vi "Main.vi"() -> ()   [LabVIEW 2015]
uses:
  <vilib>/NI/PowerElectronicsControl/BufferLogging/BufferConfig.ctl
  <vilib>/NI/PowerElectronicsControl/ScaleAndLimit/Interface/Configuration.ctl
  <vilib>/FPGAPlugInAG/sbRIO-9607/niLvFpga_Open_sbRIO-9607.vi
  <vilib>/rvi/interface/common/dynamic/niFpgaDynamicAddResources.vi
  <vilib>/FPGAPlugInAG/Dynamic/niLvFpga_Reset_Dynamic.vi
  <vilib>/FPGAPlugInAG/Dynamic/niLvFpga_Run_Dynamic.vi
  <vilib>/Utility/error.llb/Error Cluster From Error Code.vi
  <vilib>/rvi/errors/niLvFpgaAdjustHostInterfaceError.vi
  <vilib>/rvi/interface/nirviOpenFPGA/nirviOpenFPGA.xnode
  FPGA Bitfiles/BaseApplication_FPGATarget_Firmware_DvSj-lU7Yzc.lvbitx
  FPGA/Firmware.vi
  <vilib>/rvi/interface/nirviMethod/nirviMethod.xnode
  <vilib>/rvi/interface/nirviReadWriteControl/nirviReadWriteControl.xnode
  <instrlib>/_niInstr/FIFO Register Bus/v1/Host/niInstr FIFO Register Bus v1 Host.lvclass
  <vilib>/NI/PowerElectronicsControl/BufferLogging/BufferLogging.lvlib
  <instrlib>/_niInstr/Instruction Framework/v1/Host/Subsystem Map/niInstr Subsystem Map v1 Host.lvclass
  <vilib>/NI/PowerElectronicsControl/ScaleAndLimit/Interface/ScaleAndLimitInterface.lvlib
  <vilib>/NI/PowerElectronicsControl/WaveformAcq/IFw_Addon/RT/WaveformTask.lvclass
  NiFpgaLv.dll
  <vilib>/rvi/interface/Simulation/niFpgaSimulationCallBeginRW.vi
panel:
  out "AI Limits":string
  in  "UI Update Rate(s)":dbl=5.0 format="%#_13g"
  in  "TriggerLog":bool
  out "Waveforms":sgl[][](graph)
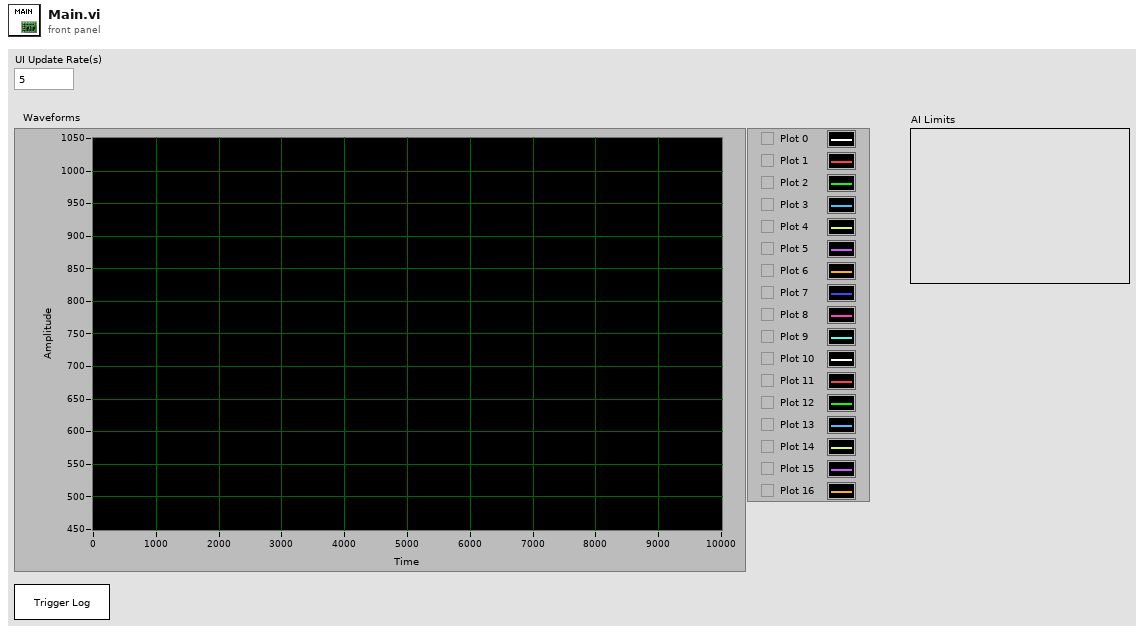
[diagram p1: front panel]
types:
  T1 = cluster{"Channel Name":string, "Sensitivity mV_EU":dbl, "EU":string, "dB Ref EU":dbl}
  T2 = typedef "BufferLogging.lvlib/BufferConfig.ctl" = cluster{"Channels":string[], "pretriggerTime_sec":dbl, "posttriggerTime_sec":dbl, "BlockSizePerChannel":i32, "SampleRate_Hz":dbl, "decimation factor":i32, "logDirectory":path, "logPrefix":string, "max files":i32}
  T3 = typedef "ScaleAndLimitInterface.lvlib/Configuration.ctl" = cluster{"Name":string, "M":dbl, "B":i16, "HighLimit":dbl, "LowLimit":dbl, "LimitsEnabled":bool}
  T4 = cluster{"Channel Name":string, "Sensitivity mV_EU":dbl, "EU":string, "dB Ref EU":dbl}[]
  T5 = typedef "BufferLogging.lvlib/Buffers.ctl" = cluster{"Channels":string[], "PosttriggerBuffer":refnum<queue>, "PretriggerBuffer":refnum<queue>, "BlockSizePerChannel":i32, " logging semaphore":T6, "Log refnum":refnum<k34>, "snapshotBuffer":refnum<data-value>, "logDirectory":path, "logPrefix":string, "decimation factor":i32, "max files":i32, "SampleRate":dbl}
  T6 = typedef "Semaphore RefNum" = refnum<k1>
  T7 = typedef "ScaleAndLimitInterface.lvlib/Interface.ctl" = cluster{"instruction target":refnum<class "niInstr Instruction Target v1 Host.lvclass">, "ScalingAndLimitsContext":refnum<class "niInstr Instruction Framework Context v1 Host.lvclass">, "Configuration":T3[]}
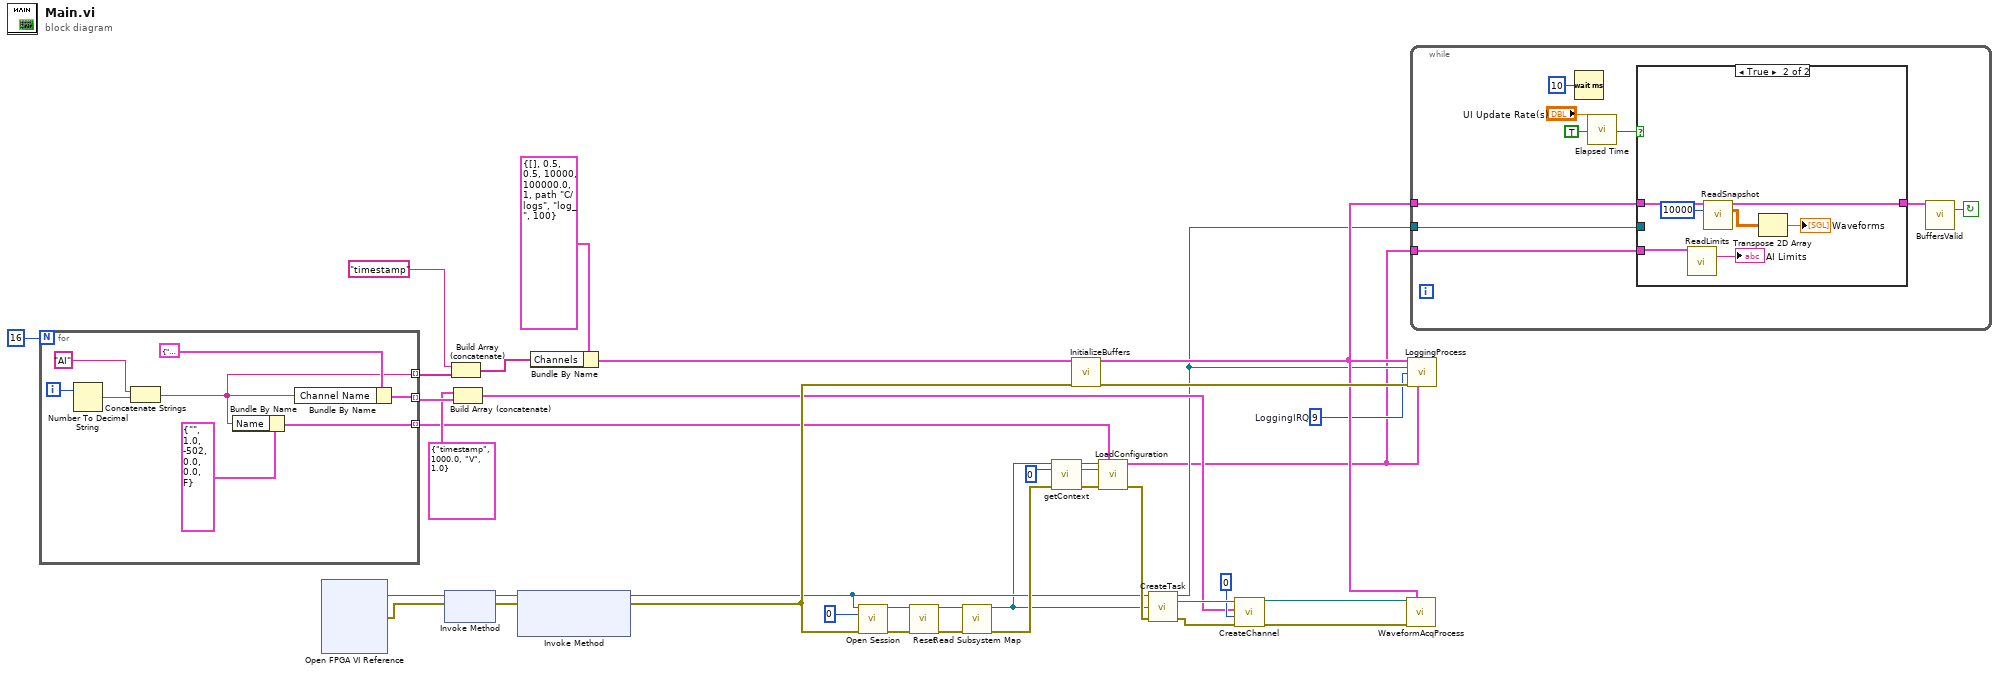
[diagram p0: block diagram]
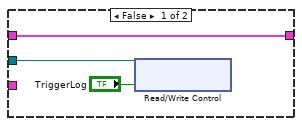
[diagram p2: hidden frame]
diagram:
  w2 = 9  # LoggingIRQ
  n1 = for {
    N: 16 -> [_]
    tunnel: [w40] -> w30 mode=indexing
    tunnel: [w42] -> w32 mode=indexing
    tunnel: [w39] -> w9 mode=indexing
    i -> [w46]
    n2 = Number To Decimal String(number=w46) -> (decimal integer string=w45:string)  [unwired: 1 in]
    n3 = Concatenate Strings("AI", w45) -> (w40:string)
    n4 = Bundle By Name(cluster=T3 {"Name"="", "M"=1.0, "B"=-502, "HighLimit"=0.0, "LowLimit"=0.0, "LimitsEnabled"=FALSE} ("Configuration"), "Name"=w40) -> (w39:T3)
    n5 = Bundle By Name(cluster=T1 {"Channel Name"="Untitled", "Sensitivity mV_EU"=1000.0, "EU"="V", "dB Ref EU"=1.0} ("Channel Info 2"), "Channel Name"=w40) -> (w42:T1)
  }
  n6 = xnode "Open FPGA VI Reference"() -> ("FPGA VI Reference Out"=w37:refnum<k20>, "error out"=w36:errorcluster)  [unwired: 2 in]
  n7 = xnode "Invoke Method"("FPGA VI Reference In"=w37, "error in"=w36) -> ("FPGA VI Reference Out"=w38:refnum<k20>, "error out"=w21:errorcluster)
  n8 = Build Array (concatenate)("timestamp", w30) -> (w28:string[])
  n9 = Build Array (concatenate)(T1 {"Channel Name"="timestamp", "Sensitivity mV_EU"=1000.0, "EU"="V", "dB Ref EU"=1.0} ("Channel Info 2"), w32) -> (w10:T4)
  n10 = xnode "Invoke Method"("FPGA VI Reference In"=w38, "error in"=w21) -> ("FPGA VI Reference Out"=w5:refnum<k20>, "error out"=w11:errorcluster)  [unwired: 1 in]
  n11 = Bundle By Name(cluster=T2 {"Channels"=[], "pretriggerTime_sec"=0.5, "posttriggerTime_sec"=0.5, "BlockSizePerChannel"=10000, "SampleRate_Hz"=100000.0, "decimation factor"=1, "logDirectory"=path "C:/logs", "logPrefix"="log_", "max files"=100} ("BufferConfig"), "Channels"=w28) -> (w34:T2)
  n12 = call <instrlib>:"Open Session.vi"("fpga ref"=w5, "bus instance"=u32 0, "error in"=w11) -> ("session out"=w24:refnum<class "niInstr FIFO Register Bus v1 Host.lvclass">, "error out"=w26:errorcluster)  [unwired: 11 in]
  n13 = call-dynamic "Reset.vi"("session in"=w24, "error in"=w26) -> ("session out"=w23:refnum<class "niInstr FIFO Register Bus v1 Host.lvclass">, "error out"=w22:errorcluster)  [unwired: 12 in]
  n14 = call <instrlib>:"Read Subsystem Map.vi"("instruction target in"=w23, "error in"=w22) -> ("instruction target out"=w4:refnum<class "niInstr FIFO Register Bus v1 Host.lvclass">, "error out"=w12:errorcluster)  [unwired: 11 in, 1 out]
  n15 = call <vilib>:"getContext.vi"("session in"=w4, "instance"=u8 0, "error in"=w12) -> ("session out"=w18:refnum<class "niInstr FIFO Register Bus v1 Host.lvclass">, "ScalingAndLimitsContext"=w20:refnum<class "niInstr Instruction Framework Context v1 Host.lvclass">, "error out"=w16:errorcluster)  [unwired: 10 in]
  n16 = call <vilib>:"InitializeBuffers.vi"("BufferConfig"=w34, "error in (no error)"=w11) -> ("Buffers"=w8:T5, "error out"=w27:errorcluster)  [unwired: 12 in]
  n17 = call <vilib>:"LoadConfiguration.vi"("instruction target in"=w18, "Configuration"=w9, "ScalingAndLimitsContext"=w20, "error in (no error)"=w16) -> ("Interface"=w1:T7, "error out"=w19:errorcluster)  [unwired: 10 in]
  n18 = call <vilib>:"CreateTask.vi"("FPGA Ref in"=w5, "session in"=w4, "error in"=w19) -> ("FPGA Ref out"=w3:refnum<k20>, "Task out"=w15:refnum<class "WaveformTask.lvclass">, "error out"=w14:errorcluster)  [unwired: 9 in, 1 out]
  n19 = call <vilib>:"CreateChannel.vi"("error in"=w14, "instance"=u8 0, "Channel Info"=w10, "task in"=w15) -> ("error out"=w6:errorcluster, "Task out"=w7:refnum<class "WaveformTask.lvclass">)  [unwired: 6 in]
  n20 = call "WaveformAcqProcess.vi"("Task in"=w7, "Buffers"=w8, "error in (no error)"=w6) -> ()  [unwired: 13 in]
  n21 = call "LoggingProcess.vi"("Buffers"=w8, "FPGA Ref"=w3, "LoggingIRQ"=w2, "error in (no error)"=w27, "Interface"=w1) -> ()  [unwired: 11 in]
  n22 = while {
    tunnel: w8 -> [w55]
    tunnel: w3 -> [w48]
    tunnel: w1 -> [w47]
    stop <- w53 continue-if-true
    n23 = Wait (ms)(milliseconds to wait=u32 10) -> ()  [unwired: 1 out]
    n24 = call "Elapsed Time"("Time Target (s)"="UI Update Rate(s)", "Auto Reset"=TRUE) -> ("Time has Elapsed"=w50:bool)  [unwired: 10 in, 7 out]
    n25 = case shown="True" w50 {
      tunnel: w55 -> [w58 w65]
      tunnel: [w58 w64] -> w54
      tunnel: w48 -> [w57 _]
      tunnel: w47 -> [_ w60]
      frame False {
        n26 = xnode "Read/Write Control"("FPGA VI Reference In"=w57, "ManualTrigger"="TriggerLog") -> ()  [unwired: 1 in, 2 out]
      }
      frame True {
        n27 = call <vilib>:"ReadLimits.vi"("Interface in"=w60) -> ("Limits"=→"AI Limits":string)  [unwired: 12 in, 2 out]
        n28 = call <vilib>:"ReadSnapshot.vi"("Buffers in"=w65, "sizeOfBlock"=10000) -> ("Buffers out"=w64:T5, "snapshot"=w62:sgl[][])  [unwired: 11 in, 1 out]
        n29 = Transpose 2D Array(2D array=w62) -> (transposed array=→"Waveforms":sgl[][])
      }
    }
    n30 = call <vilib>:"BuffersValid.vi"("Buffers in"=w54) -> ("valid"=w53:bool)  [unwired: 13 in, 1 out]
  }
